vi "Num Channels.vi"(8 "error in (no error)":errorcluster, 11 "GroupAbstract in":refnum<class "GroupAbstract.lvclass">) -> (0 "error out":errorcluster, 2 "Num Channels":i32, 3 "GroupAbstract out":refnum<class "GroupAbstract.lvclass">)   [LabVIEW 2020, in "Vecto.lvlib" / "GroupAbstract.lvclass"]
uses:
  GroupAbstract.lvclass
  GroupAbstract.lvclass/GroupAbstract.ctl
  Group Config/Group Config.lvclass
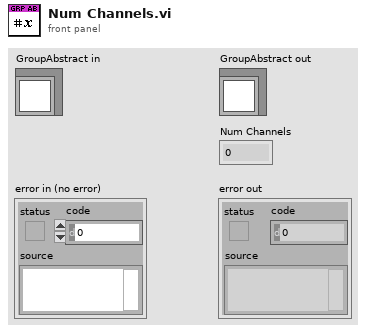
[diagram p1: front panel]
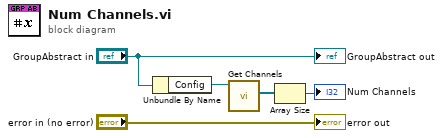
[diagram p0: block diagram]
diagram:
  n1 = Unbundle By Name("GroupAbstract in") -> ("Config"=w3:refnum<class "Group Config.lvclass">)
  n2 = call "Get Channels.vi"("Group Config in"=w3) -> ("Channels"=w2:refnum<class "Channel Config.lvclass">[])  [unwired: 8 in, 2 out]
  n3 = Array Size(array=w2) -> (size(s)=→"Num Channels":i32)
  "error out" <- "error in (no error)"
  "GroupAbstract out" <- "GroupAbstract in"
